vi "Save-FWM-Data.vi"(6 "unit":enum16{"fs", "ps", "um", "mm", "counts"}(ring), 7 "Sample Channel Units":u16(ring), 8 "Data:  FWM":dbl[][](array[numeric]), 9 "Calibrated wavelength":dbl[](array[numeric]), 10 "Delay":dbl[](array[numeric]), 11 "Temperature":dbl[](array[numeric])) -> ()   [LabVIEW 2009]
panel:
  in  "size(s) temp":i32
  in  "size(s) delay":i32
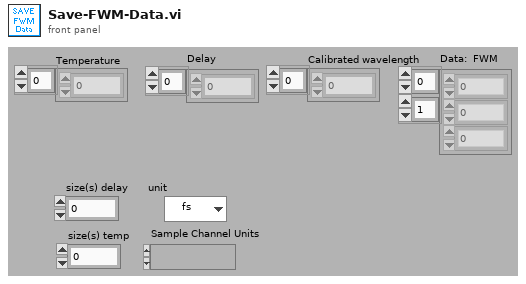
[diagram p1: front panel]
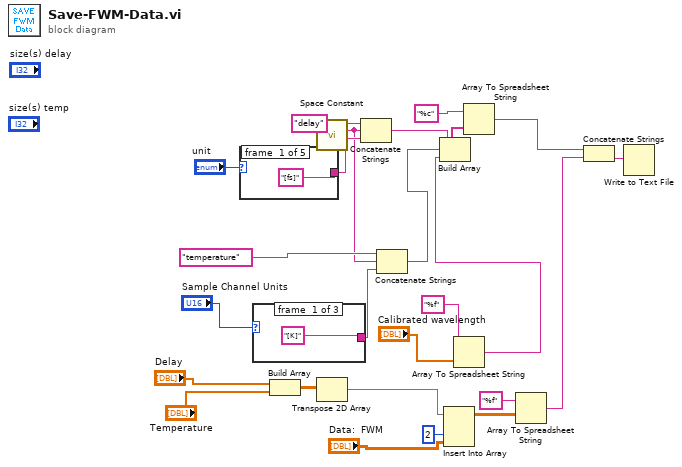
[diagram p0: block diagram]
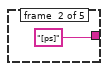
[diagram p2: hidden frame]
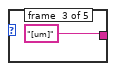
[diagram p3: hidden frame]
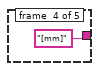
[diagram p4: hidden frame]
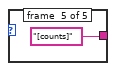
[diagram p5: hidden frame]
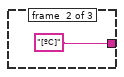
[diagram p6: hidden frame]
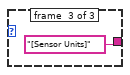
[diagram p7: hidden frame]
diagram:
  n1 = case shown="\"counts\"" "unit" {
    tunnel: ["[fs]" "[ps]" "[um]" "[mm]" "[counts]"] -> w15
    frame #0 {
    }
    frame #1 {
    }
    frame #2 {
    }
    frame #3 {
    }
    frame #4 {
    }
  }
  n2 = case shown="0, Default" "Sample Channel Units" {
    tunnel: ["[K]" "[ºC]" "[Sensor Units]"] -> w22
    frame #0 {
    }
    frame #1 {
    }
    frame #2 {
    }
  }
  n3 = Build Array("Delay", "Temperature") -> (w12:dbl[][])
  n4 = call <vilib>:"Space Constant.vi"() -> ("String"=w6:string)
  n5 = Transpose 2D Array(2D array=w12) -> (transposed array=w10:dbl[][])
  n6 = Concatenate Strings("delay", w6, w15) -> (w19:string)
  n7 = Concatenate Strings("temperature", w6, w22) -> (w7:string)
  n8 = Insert Into Array(array=w10, index (col)=2 ("disabled index (col)"), new element="Data:  FWM") -> (w8:dbl[][])  [unwired: 1 in]
  n9 = Array To Spreadsheet String(array="Calibrated wavelength", 3:"%f" ("format string")) -> (spreadsheet string=w2:string)  [unwired: 1 in]
  n10 = Build Array(w19, w7, w2) -> (w18:string[])
  n11 = Array To Spreadsheet String(array=w18, 3:"%c" ("format string")) -> (spreadsheet string=w1:string)  [unwired: 1 in]
  n12 = Array To Spreadsheet String(array=w8, 3:"%f") -> (spreadsheet string=w11:string)  [unwired: 1 in]
  n13 = Concatenate Strings(w1, w11) -> (w25:string)
  n14 = Write to Text File(text=w25) -> ()  [unwired: 3 in, 3 out]
